vi "Expanding Animation Done Callback.vi"(11 "Owner":refnum<class>) -> ()   [LabVIEW 2020, in "PicoG-Processor.lvlib" / "GVIWebProcessorApp.lvclass"]
uses:
  GVIWebProcessorApp.lvclass
  GVIWebProcessorApp.lvclass/GVIWebProcessorApp.ctl
  <vilib>/IlluminatedG/IG OOPanel/OOPanel/ArrayManager/ArrayManager.lvclass
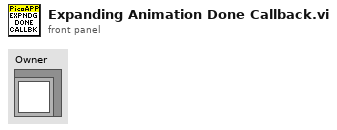
[diagram p1: front panel]
types:
  T1 = typedef "PicoG-Processor.lvlib/GVIWebProcessorApp.lvclass/Ref Data.ctl" = cluster{"hWnd":i32, "UI Refs":T2, "Collapsed":bool, "Async Anim Ref":refnum<vi>, "Expanded Bounds":T3, "Expanding":bool, "Collapsing":bool}
  T2 = typedef "PicoG-Processor.lvlib/GVIWebProcessorApp.lvclass/UI Refs.ctl" = cluster{"Main Window":refnum<vi>, "List Panel":refnum<vi>, "H Splitter":refnum<vi>, "V Splitter":refnum<vi>, "Open Project":refnum<vi>, "Project Name":refnum<vi>}
  T3 = typedef "LVRectTypeDef.ctl" = cluster{"Left":i16, "Top":i16, "Right":i16, "Bottom":i16}
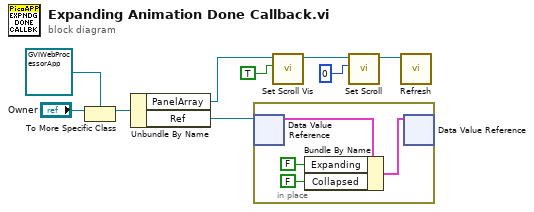
[diagram p0: block diagram]
diagram:
  n1 = To More Specific Class(target class=refnum<class "GVIWebProcessorApp.lvclass"> refnum ("PicoG-Processor:GVIWebProcessorApp.lvclass"), reference="Owner") -> (specific class reference=w7:refnum<class "GVIWebProcessorApp.lvclass">)  [unwired: 1 in, 1 out]
  n2 = Unbundle By Name(w7) -> ("PanelArray"=w5:refnum<class "ArrayManager.lvclass">, "Ref"=w8:refnum<data-value>)
  n3 = in-place {
    n4 = in-place-dvr #1(w8) -> (w13:T1)  [unwired: 1 out]
    n5 = Bundle By Name(cluster=w13, "Expanding"=FALSE ("Collapsing"), "Collapsed"=FALSE) -> (w12:T1)
    n6 = in-place-dvr #1(w12) -> ()  [unwired: 2 out]
  }
  n7 = call <vilib>:"Set Scroll Vis.vi"("Scroll Visible"=TRUE, "ArrayManager in"=w5) -> ("ArrayManager out"=w4:refnum<class "ArrayManager.lvclass">)  [unwired: 8 in, 1 out]
  n8 = call <vilib>:"Set Scroll.vi"("Position"=0, "ArrayManager in"=w4) -> ("ArrayManager out"=w1:refnum<class "ArrayManager.lvclass">)  [unwired: 8 in, 1 out]
  n9 = call <vilib>:"Refresh.vi"("ArrayManager in"=w1) -> ()  [unwired: 9 in, 2 out]
